vi "Create Auto Config.vi"   [LabVIEW 2017]
uses:
  Routines and Block Data.ctl
  2018_Trobots_5013_Robot/Support Code/Blocks.ctl
types:
  T1 = typedef "Routines and Block Data.ctl" = cluster{"Routines":T2[][]}
  T2 = typedef "Blocks.ctl" = enum16{"", "Wait", "Far to L1", "L1 to End Switch 1", "End Switch 1 to C1", "End Cube to C1", "C1 to Diag Scale 1", "C1 to C3", "C3 to C4", "Diag Scale to C1", "C3 to End Switch 2", "C4 to Diag Scale 2", "C3 to Cube&Switch", "Middle to Front S2", "Middle to Front S1", "Front S1 to Line 1", "Front S2 to Line 2", "End Switch 1 to End Cube", "Line 1 to C1"}
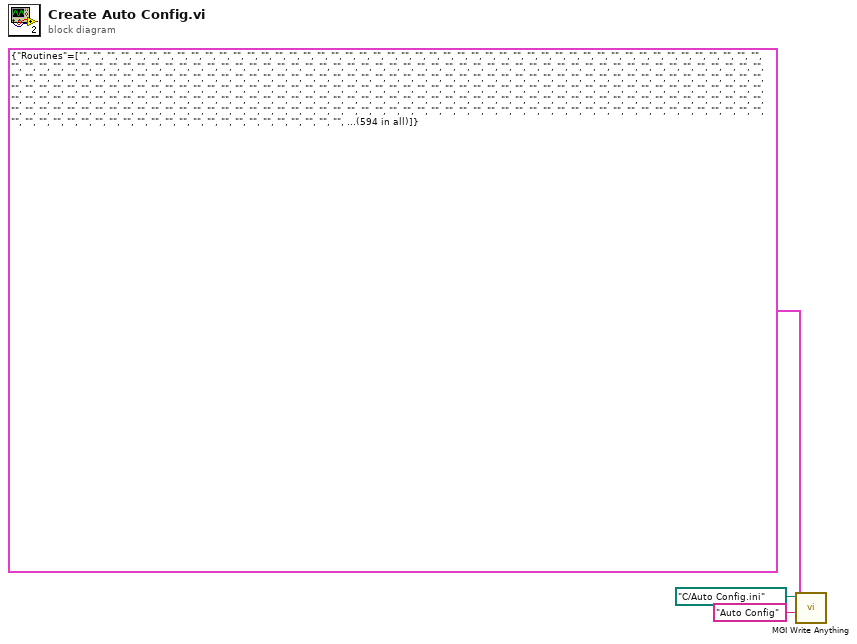
[diagram p0: block diagram]
diagram:
  n1 = call <userlib>:"MGI Write Anything.vi"("Section Name (Name of \"Anything\")"="Auto Config" ("Section Name (Name of \"Anything\")"), "Anything"=T1 {"Routines"=[[enum."", enum."", enum."", enum."", enum."", enum."", enum."", enum."", enum."", enum."", enum."", enum."", enum."", enum."", enum."", enum."", enum."", enum."", enum."", enum."", enum."", enum.""], [enum."", enum."", enum."", enum."", enum."", enum."", enum."", enum."", enum."", enum."", enum."", enum."", enum."", enum."", enum."", enum."", enum."", enum."", enum."", enum."", enum."", enum.""], [enum."", enum."", enum."", enum."", enum."", enum."", enum."", enum."", enum."", enum."", enum."", enum."", enum."", enum."", enum."", enum."", enum."", enum."", enum."", enum."", enum."", enum.""], [enum."", enum."", enum."", enum."", enum."", enum."", enum."", enum."", enum."", enum."", enum."", enum."", enum."", enum."", enum."", enum."", enum."", enum."", enum."", enum."", enum."", enum.""], [enum."", enum."", enum."", enum."", enum."", enum."", enum."", enum."", enum."", enum."", enum."", enum."", enum."", enum."", enum."", enum."", enum."", enum."", enum."", enum."", enum."", enum.""], [enum."", enum."", enum."", enum."", enum."", enum."", enum."", enum."", enum."", enum."", enum."", enum."", enum."", enum."", enum."", enum."", enum."", enum."", enum."", enum."", enum."", enum.""], [enum."", enum."", enum."", enum."", enum."", enum."", enum."", enum."", enum."", enum."", enum."", enum."", enum."", enum."", enum."", enum."", enum."", enum."", enum."", enum."", enum."", enum.""], [enum."", enum."", enum."", enum."", enum."", enum."", enum."", enum."", enum."", enum."", enum."", enum."", enum."", enum."", enum."", enum."", enum."", enum."", enum."", enum."", enum."", enum.""], [enum."", enum."", enum."", enum."", enum."", enum."", enum."", enum."", enum."", enum."", enum."", enum."", enum."", enum."", enum."", enum."", enum."", enum."", enum."", enum."", enum."", enum.""], [enum."", enum."", enum."", enum."", enum."", enum."", enum."", enum."", enum."", enum."", enum."", enum."", enum."", enum."", enum."", enum."", enum."", enum."", enum."", enum."", enum."", enum.""], [enum."", enum."", enum."", enum."", enum."", enum."", enum."", enum."", enum."", enum."", enum."", enum."", enum."", enum."", enum."", enum."", enum."", enum."", enum."", enum."", enum."", enum.""], [enum."", enum."", enum."", enum."", enum."", enum."", enum."", enum."", enum."", enum."", enum."", enum."", enum."", enum."", enum."", enum."", enum."", enum."", enum."", enum."", enum."", enum.""], [enum."", enum."", enum."", enum."", enum."", enum."", enum."", enum."", enum."", enum."", enum."", enum."", enum."", enum."", enum."", enum."", enum."", enum."", enum."", enum."", enum."", enum.""], [enum."", enum."", enum."", enum."", enum."", enum."", enum."", enum."", enum."", enum."", enum."", enum."", enum."", enum."", enum."", enum."", enum."", enum."", enum."", enum."", enum."", enum.""], [enum."", enum."", enum."", enum."", enum."", enum."", enum."", enum."", enum."", enum."", enum."", enum."", enum."", enum."", enum."", enum."", enum."", enum."", enum."", enum."", enum."", enum.""], [enum."", enum."", enum."", enum."", enum."", enum."", enum."", enum."", enum."", enum."", enum."", enum."", enum."", enum."", enum."", enum."", enum."", enum."", enum."", enum."", enum."", enum.""], [enum."", enum."", enum."", enum."", enum."", enum."", enum."", enum."", enum."", enum."", enum."", enum."", enum."", enum."", enum."", enum."", enum."", enum."", enum."", enum."", enum."", enum.""], [enum."", enum."", enum."", enum."", enum."", enum."", enum."", enum."", enum."", enum."", enum."", enum."", enum."", enum."", enum."", enum."", enum."", enum."", enum."", enum."", enum."", enum.""], [enum."", enum."", enum."", enum."", enum."", enum."", enum."", enum."", enum."", enum."", enum."", enum."", enum."", enum."", enum."", enum."", enum."", enum."", enum."", enum."", enum."", enum.""], [enum."", enum."", enum."", enum."", enum."", enum."", enum."", enum."", enum."", enum."", enum."", enum."", enum."", enum."", enum."", enum."", enum."", enum."", enum."", enum."", enum."", enum.""], [enum."", enum."", enum."", enum."", enum."", enum."", enum."", enum."", enum."", enum."", enum."", enum."", enum."", enum."", enum."", enum."", enum."", enum."", enum."", enum."", enum."", enum.""], [enum."", enum."", enum."", enum."", enum."", enum."", enum."", enum."", enum."", enum."", enum."", enum."", enum."", enum."", enum."", enum."", enum."", enum."", enum."", enum."", enum."", enum.""], [enum."", enum."", enum."", enum."", enum."", enum."", enum."", enum."", enum."", enum."", enum."", enum."", enum."", enum."", enum."", enum."", enum."", enum."", enum."", enum."", enum."", enum.""], [enum."", enum."", enum."", enum."", enum."", enum."", enum."", enum."", enum."", enum."", enum."", enum."", enum."", enum."", enum."", enum."", enum."", enum."", enum."", enum."", enum."", enum.""], [enum."", enum."", enum."", enum."", enum."", enum."", enum."", enum."", enum."", enum."", enum."", enum."", enum."", enum."", enum."", enum."", enum."", enum."", enum."", enum."", enum."", enum.""], [enum."", enum."", enum."", enum."", enum."", enum."", enum."", enum."", enum."", enum."", enum."", enum."", enum."", enum."", enum."", enum."", enum."", enum."", enum."", enum."", enum."", enum.""], [enum."", enum."", enum."", enum."", enum."", enum."", enum."", enum."", enum."", enum."", enum."", enum."", enum."", enum."", enum."", enum."", enum."", enum."", enum."", enum."", enum."", enum.""]]} ("Routines and Block Data"), "Path (dialog)"=path "C:/Auto Config.ini") -> ()  [unwired: 6 in, 3 out]
